vi "EventProgressToEventCount.vi"(9 "CurrentEntry":string, 10 "EventProgressDataInput":string[][](array[string])) -> (2 "EventCount":i32)   [LabVIEW 2020]
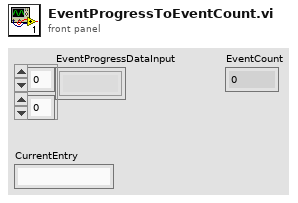
[diagram p1: front panel]
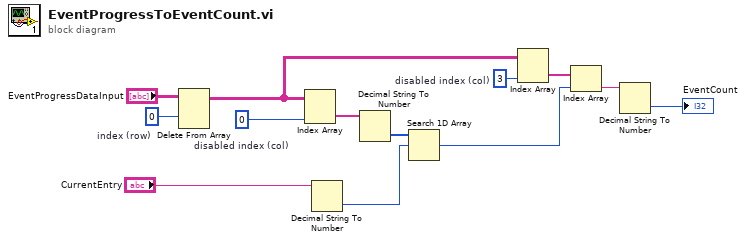
[diagram p0: block diagram]
diagram:
  w1 = 0  # index (row)
  w9 = 3  # disabled index (col)
  w3 = 0  # disabled index (col)
  n1 = Delete From Array "Delete From Array"(array="EventProgressDataInput", index (row)=w1) -> (array with subset deleted=w8:string[][])  [unwired: 2 in, 1 out]
  n2 = Index Array "Index Array"(array=w8, index (col)=w3) -> (element=w4:string[])  [unwired: 1 in]
  n3 = Decimal String To Number(string="CurrentEntry") -> (number=w7:i32)  [unwired: 2 in, 1 out]
  n4 = Decimal String To Number(string=w4) -> (number=w5:i32[])  [unwired: 2 in, 1 out]
  n5 = Search 1D Array(1D array=w5, element=w7) -> (index of element=w11:i32)  [unwired: 1 in]
  n6 = Index Array "Index Array"(array=w8, index (col)=w9) -> (element=w10:string[])  [unwired: 1 in]
  n7 = Index Array "Index Array"(array=w10, index=w11) -> (element=w12:string)
  n8 = Decimal String To Number(string=w12) -> (number=→"EventCount":i32)  [unwired: 2 in, 1 out]
